vi "Untitled 1.vi"() -> ()   [LabVIEW 2015]
uses:
  Setting_Control_Main Action.ctl
  <vilib>/Utility/miscctls.llb/LVPositionTypeDef.ctl
  <vilib>/ptbypt/NI_PtbyPt.lvlib
panel:
  in  "Boolean":bool
  out "Array":T1[](array[typedef])=[enum."二、動作-單次取像", enum."三、動作-連續取像"]
  out "Setting Action":T1
  in  "Tab Control":enum32{"設定", "Match參數", "找邊參數", "找圓參數"}(tab)
  in  "功能選擇":enum16{"Pattern", "Match", "找邊", "找圓"}(ring)
  in  "匯入圖片":bool
  in  "確認檢測項目":bool
  in  "Cluster":T2
  out "Pattern":T3(plugin-control)
  out "Image":T3(plugin-control)
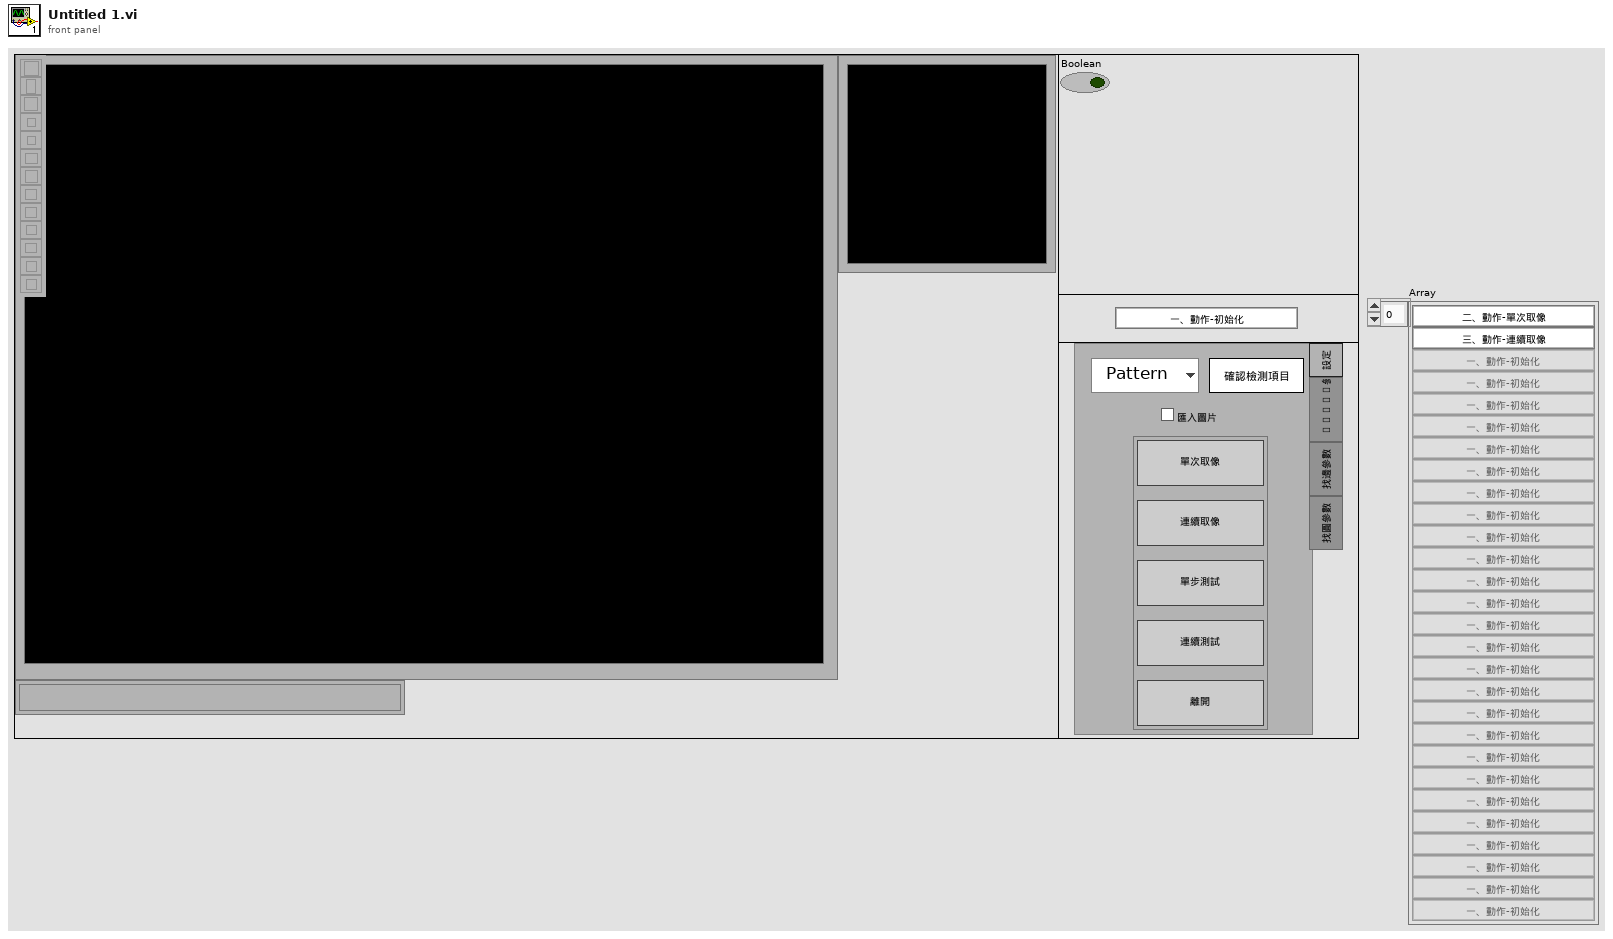
[diagram p1: front panel]
types:
  T1 = typedef "Setting_Control_Main Action.ctl" = enum16{"一、動作-初始化", "二、動作-單次取像", "三、動作-連續取像", "四、動作-單步測試", "五、動作-連續測試", "六、動作-離開", "1.0 功能-IO控制", "       1.1 IO-初始化", "       1.2 Set Point(EOT On)", "       1.3Set Point(EOT Off)", "       1.4Get Point(SOT)", "2.0功能-相機控制", "       2.1相機-初始化", "       2.2相機-取像", "       2.3相機-關閉", "3.0功能-影像控制", "       3.1影像-初始化", "       3.2影像-更新影像", "       3.3影像-儲存影像", "4.0功能-檢測", "       4.1檢測-初始化", "      4.2浪代-浪代", "             4.2.1浪代-Pattern", "             4.2.2浪代-Match", "             4.2.3檢測-找邊", "             4.2.4檢測-找圓", "5.0功能-檔案", "       5.1檔案-初始化", "       5.2檔案-儲存檔案", "       5.3檔案-開啟檔案", "       5.4檔案-匯入檔案", "6.0 錯誤", "7.0等待", "       7.1等待(計算時間)", "8.0離開", "9.0功能-機台驗證", "      9.1機台驗證-初始化", "      9.2機台驗證-檢測", "10.0對話視窗", "11.光源控制", "       11.1光源控制-初始化", "       11.2光源控制-光源開啟", "       11.3光源控制-光源關閉", "       11.4光源控制-通訊關閉"}
  T2 = cluster{"二、動作-單次取像":bool, "三、動作-連續取像":bool, "四、動作-單步測試":bool, "五、動作-連續測試":bool, "六、動作-離開":bool}
  T3 = typedef "IMAQ Image.ctl" = refnum<image>
  T4 = typedef "LVPositionTypeDef.ctl" = cluster{"Left":i32, "Top":i32}
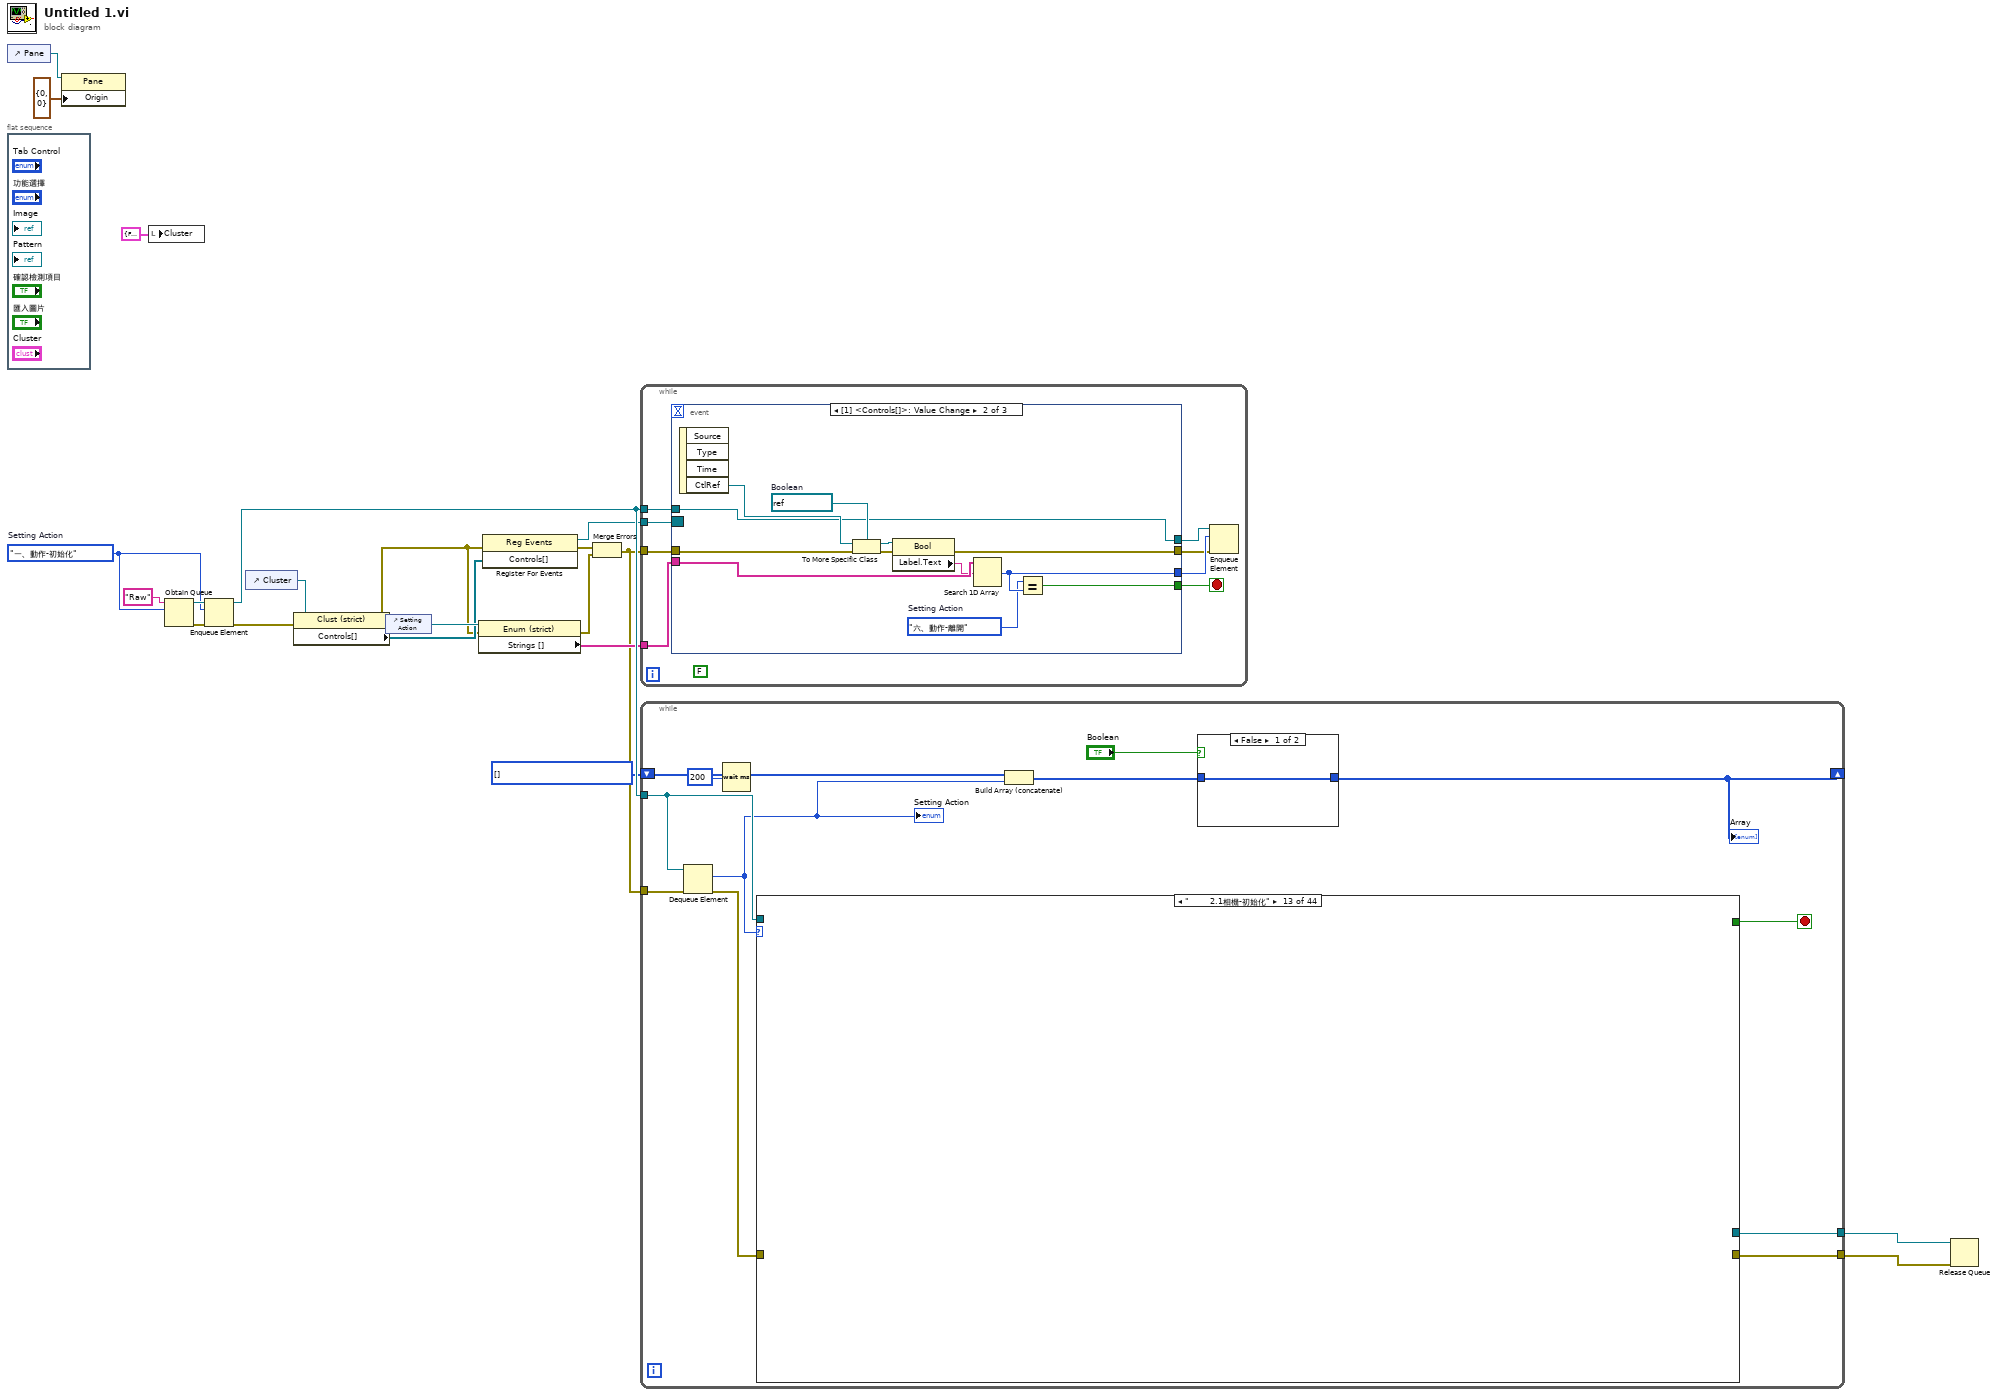
[diagram p0: block diagram]
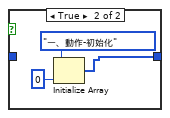
[diagram p2: hidden frame]
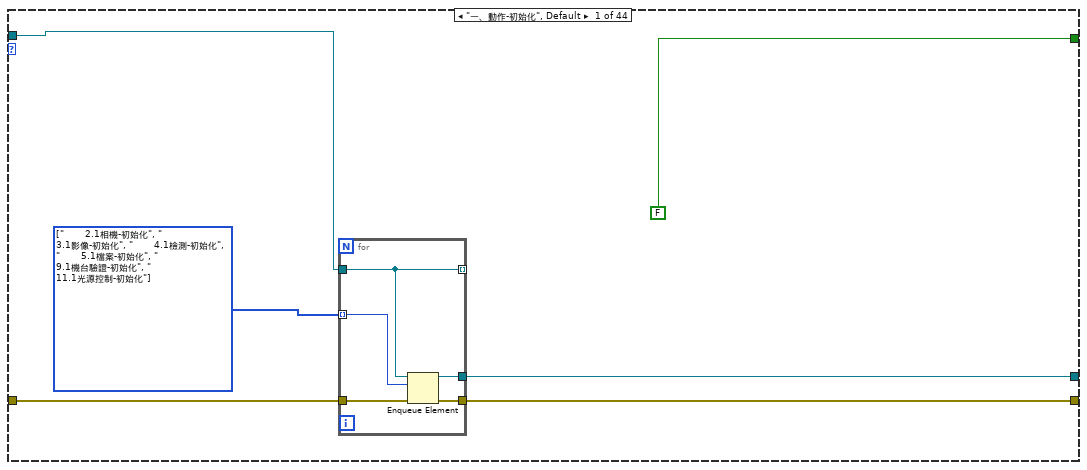
[diagram p3: hidden frame]
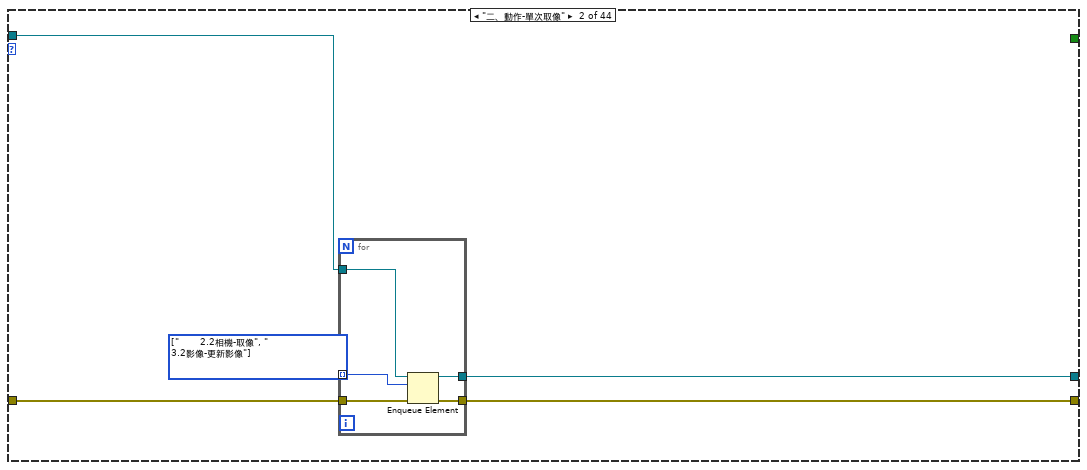
[diagram p4: hidden frame]
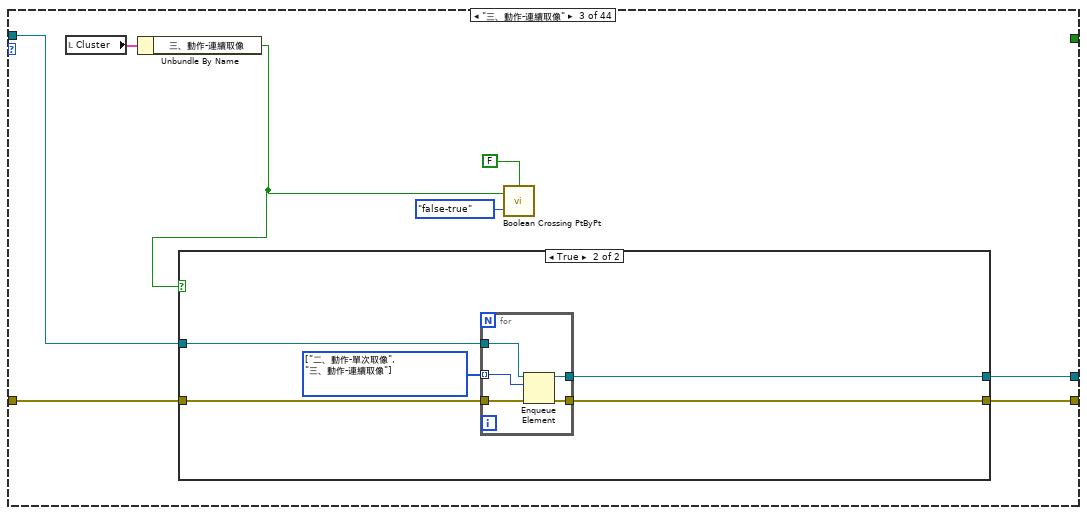
[diagram p5: hidden frame]
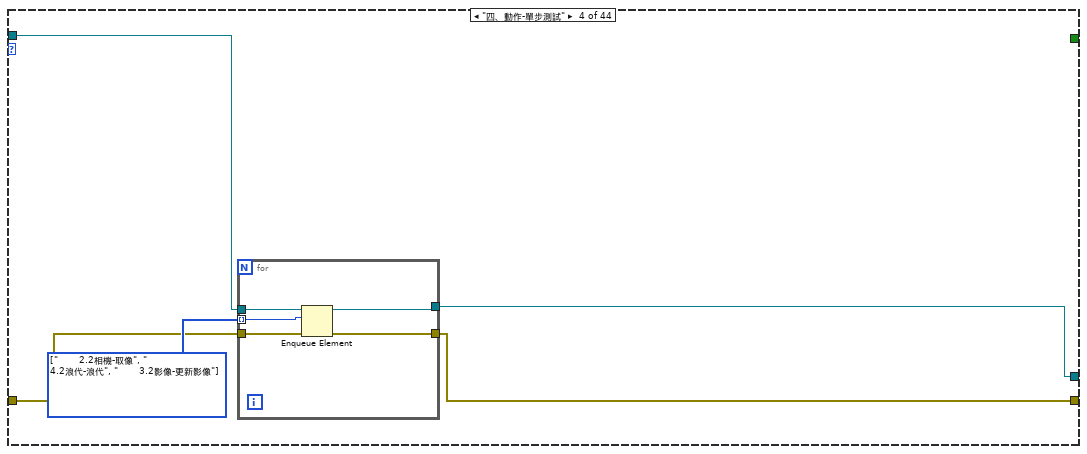
[diagram p7: hidden frame]
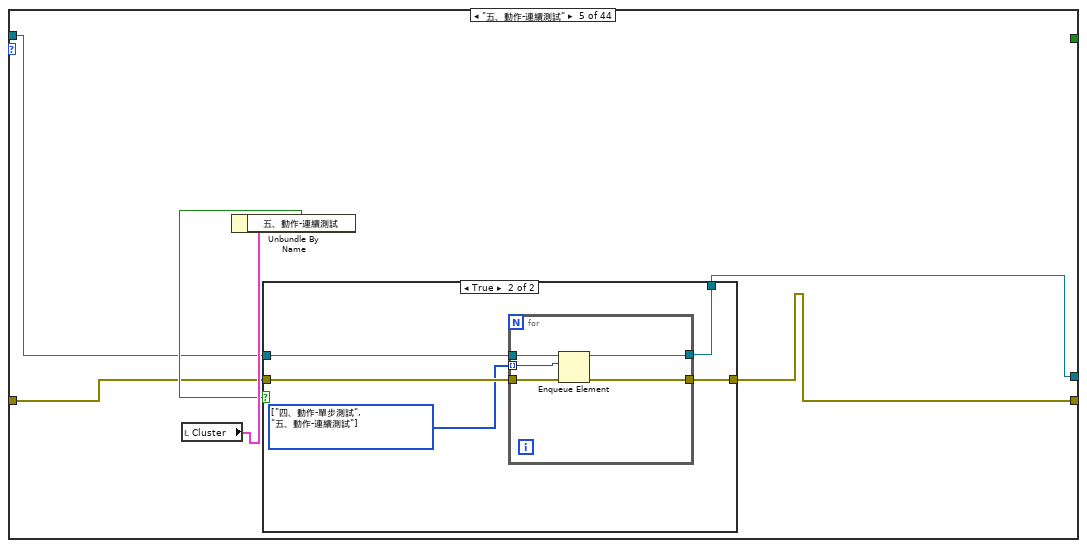
[diagram p8: hidden frame]
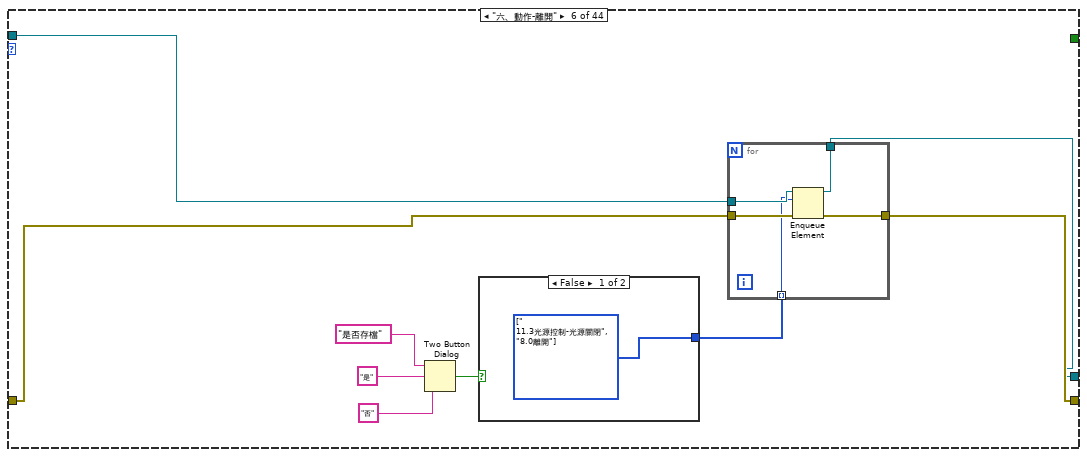
[diagram p10: hidden frame]
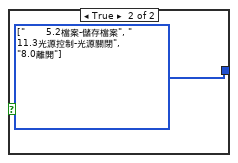
[diagram p11: hidden frame]
diagram:
  w2 = T1[] [] items=["一、動作-初始化", "二、動作-單次取像", "三、動作-連續取像", "四、動作-單步測試", "五、動作-連續測試", "六、動作-離開", "1.0 功能-IO控制", "       1.1 IO-初始化", "       1.2 Set Point(EOT On)", "       1.3Set Point(EOT Off)", "       1.4Get Point(SOT)", "2.0功能-相機控制", "       2.1相機-初始化", "       2.2相機-取像", "       2.3相機-關閉", "3.0功能-影像控制", "       3.1影像-初始化", "       3.2影像-更新影像", "       3.3影像-儲存影像", "4.0功能-檢測", "       4.1檢測-初始化", "      4.2浪代-浪代", "             4.2.1浪代-Pattern", "             4.2.2浪代-Match", "             4.2.3檢測-找邊", "             4.2.4檢測-找圓", "5.0功能-檔案", "       5.1檔案-初始化", "       5.2檔案-儲存檔案", "       5.3檔案-開啟檔案", "       5.4檔案-匯入檔案", "6.0 錯誤", "7.0等待", "       7.1等待(計算時間)", "8.0離開", "9.0功能-機台驗證", "      9.1機台驗證-初始化", "      9.2機台驗證-檢測", "10.0對話視窗", "11.光源控制", "       11.1光源控制-初始化", "       11.2光源控制-光源開啟", "       11.3光源控制-光源關閉", "       11.4光源控制-通訊關閉"]
  w11 = Setting_Control_Main_Action."一、動作-初始化"  # Setting Action
  n1 = control-ref of="Pane"() -> (w13:refnum<vi>)
  n2 = flat-sequence {
    frame #0 {
    }
  }
  n3 = property class="Pane"(reference=w13, "Origin"=T4 {"Left"=0, "Top"=0} ("Position")) -> ()  [unwired: 1 in, 2 out]
  n4 = local write "Cluster"(T2 {"二、動作-單次取像"=FALSE, "三、動作-連續取像"=FALSE, "四、動作-單步測試"=FALSE, "五、動作-連續測試"=FALSE, "六、動作-離開"=FALSE} ("Cluster")) -> ()
  n5 = Obtain Queue(name (unnamed)="Raw", element data type=w11) -> (queue out=w21:refnum<queue>, error out=w10:errorcluster)  [unwired: 3 in, 1 out]
  n6 = Enqueue Element(queue=w21, element=w11, error in (no error)=w10) -> (queue out=w19:refnum<queue>, error out=w9:errorcluster)  [unwired: 1 in, 1 out]
  n7 = control-ref of="Cluster"() -> (w15:refnum<vi>)
  n8 = property class="Clust (strict)"(reference=w15, error in=w9) -> (error out=w8:errorcluster, "Controls[]"=w14:refnum<vi>[])  [unwired: 1 out]
  n9 = control-ref of="Setting Action"() -> (w17:refnum<vi>)
  n10 = property class="Enum (strict)"(reference=w17, error in=w8) -> (error out=w6:errorcluster, "Strings []"=w16:string[])  [unwired: 1 out]
  n11 = register-events(error in=w8, w14) -> (reference out=w18:refnum<event-registration>, error out=w7:errorcluster)  [unwired: 1 in]
  n12 = Merge Errors(w7, w6) -> (w5:errorcluster)
  n13 = while {
    tunnel: w19 -> [w29]
    tunnel: w18 -> [w28]
    tunnel: w16 -> [w27]
    tunnel: w5 -> [w23]
    stop <- w26 stop-if-true
    (unwired) FALSE
    n14 = event shown="[1] <Controls[]>: Value Change" {
      selector: w28 -> [_ _ _]
      dyn-events: _ -> [_ _ _]
      timeout: _ -> [_ _ _]
      tunnel: [w31 w37 w45] -> w25
      tunnel: w29 -> [w31 w37 w47]
      tunnel: w27 -> [_ w40 _]
      tunnel: [_ w38 _] -> w26
      tunnel: [_ w36 w46] -> w24
      tunnel: w23 -> [w30 w34 w44]
      tunnel: [w30 w32 _] -> w22
      event Timeout {
        n15 = event-data() -> ()  [unwired: 1 in, 3 out]
      }
      event Value Change {
        w35 = Setting_Control_Main_Action."六、動作-離開"  # Setting Action
        w43 = refnum<vi> refnum  # Boolean
        n16 = event-data() -> ("CtlRef"=w41:refnum<vi>)  [unwired: 1 in, 3 out]
        n17 = To More Specific Class(target class=w43, reference=w41, error in=w34) -> (specific class reference=w42:refnum<vi>, error out=w33:errorcluster)
        n18 = property class="Bool"(reference=w42, error in=w33) -> (error out=w32:errorcluster, "Label.Text"=w39:string)  [unwired: 1 out]
        n19 = Search 1D Array(1D array=w40, element=w39) -> (index of element=w36:i32)  [unwired: 1 in]
        n20 = Equal?(x=w35, y=w36) -> (x = y?=w38:bool)
      }
      event "確認檢測項目": Value Change {
        n21 = event-data() -> ()  [unwired: 1 in, 4 out]
        n22 = local read "功能選擇"() -> (w48:enum16{"Pattern", "Match", "找邊", "找圓"})
        n23 = case shown="\"Match\"" w48 {
          tunnel: w47 -> [w51 w54 w57 w60]
          tunnel: [w51 w54 w57 w60] -> w45
          tunnel: w44 -> [w50 w53 w56 w59]
          tunnel: [w50 w53 w56 w59] -> _
          tunnel: [Setting_Control_Main_Action."             4.2.1浪代-Pattern" ("Set action") Setting_Control_Main_Action."             4.2.2浪代-Match" ("Set action") Setting_Control_Main_Action."             4.2.3檢測-找邊" ("Set action") Setting_Control_Main_Action."             4.2.4檢測-找圓" ("Set action")] -> w46
          frame "Pattern", Default {
          }
          frame "Match" {
          }
          frame "找邊" {
          }
          frame "找圓" {
          }
        }
      }
    }
    n24 = Enqueue Element(queue=w25, element=w24, error in (no error)=w22) -> ()  [unwired: 1 in, 3 out]
  }
  n25 = while {
    tunnel: w19 -> [w69]
    tunnel: w5 -> [w70]
    tunnel: [w61] -> w4
    tunnel: [w67] -> w3
    shift-right: [w62] -> _
    shift-left: w2 -> [w65]
    stop <- w72 stop-if-true
    n26 = Dequeue Element(queue=w69, error in (no error)=w70) -> (element=w66:T1, error out=w68:errorcluster)  [unwired: 1 in, 2 out]
    "Setting Action" <- w66
    n27 = Wait (ms)(milliseconds to wait=u32 200) -> ()  [unwired: 1 out]
    n28 = case shown="\"       2.1相機-初始化\"" w66 {
      tunnel: [FALSE _ _ _ _ _ _ _ _ _ _ _ _ _ _ _ _ _ _ _ _ _ _ _ _ _ _ _ _ _ _ _ _ _ TRUE _ _ _ _ _ _ _ _ _] -> w72
      tunnel: [w81 w89 w102 w118 w128 w146 _ _ _ _ _ _ _ _ _ _ _ _ _ _ _ _ _ _ _ _ _ _ _ _ _ _ _ _ _ _ _ _ _ _ _ _ _ _] -> w61
      tunnel: w69 -> [w80 w91 w105 w121 w131 w149 _ _ _ _ _ _ _ _ _ _ _ _ _ _ _ _ _ _ _ _ _ _ _ _ _ _ _ _ _ _ _ _ _ _ _ _ _ _]
      tunnel: w68 -> [w79 w90 w103 w120 w130 w148 _ _ _ _ _ _ _ _ _ _ _ _ _ _ _ _ _ _ _ _ _ _ _ _ _ _ _ _ _ _ _ _ _ _ _ _ _ _]
      tunnel: [w77 w88 w104 w119 w129 w147 _ _ _ _ _ _ _ _ _ _ _ _ _ _ _ _ _ _ _ _ _ _ _ _ _ _ _ _ _ _ _ _ _ _ _ _ _ _] -> w67
      frame "一、動作-初始化", Default {
        w78 = T1[] [enum."       2.1相機-初始化", enum."       3.1影像-初始化", enum."       4.1檢測-初始化", enum."       5.1檔案-初始化", enum."      9.1機台驗證-初始化", enum."       11.1光源控制-初始化"] items=["一、動作-初始化", "二、動作-單次取像", "三、動作-連續取像", "四、動作-單步測試", "五、動作-連續測試", "六、動作-離開", "1.0 功能-IO控制", "       1.1 IO-初始化", "       1.2 Set Point(EOT On)", "       1.3Set Point(EOT Off)", "       1.4Get Point(SOT)", "2.0功能-相機控制", "       2.1相機-初始化", "       2.2相機-取像", "       2.3相機-關閉", "3.0功能-影像控制", "       3.1影像-初始化", "       3.2影像-更新影像", "       3.3影像-儲存影像", "4.0功能-檢測", "       4.1檢測-初始化", "      4.2浪代-浪代", "             4.2.1浪代-Pattern", "             4.2.2浪代-Match", "             4.2.3檢測-找邊", "             4.2.4檢測-找圓", "5.0功能-檔案", "       5.1檔案-初始化", "       5.2檔案-儲存檔案", "       5.3檔案-開啟檔案", "       5.4檔案-匯入檔案", "6.0 錯誤", "7.0等待", "       7.1等待(計算時間)", "8.0離開", "9.0功能-機台驗證", "      9.1機台驗證-初始化", "      9.2機台驗證-檢測", "10.0對話視窗", "11.光源控制", "       11.1光源控制-初始化", "       11.2光源控制-光源開啟", "       11.3光源控制-光源關閉", "       11.4光源控制-通訊關閉"]
        n29 = for {
          tunnel: [w83] -> _ mode=indexing
          tunnel: w79 -> [w87]
          tunnel: [w86] -> w77
          tunnel: [w85] -> w81
          tunnel: w78 -> [w84] mode=indexing
          tunnel: w80 -> [w83]
          n30 = Enqueue Element(queue=w83, element=w84, error in (no error)=w87) -> (queue out=w85:refnum<queue>, error out=w86:errorcluster)  [unwired: 1 in, 1 out]
        }
      }
      frame "二、動作-單次取像" {
        w92 = T1[] [enum."       2.2相機-取像", enum."       3.2影像-更新影像"] items=["一、動作-初始化", "二、動作-單次取像", "三、動作-連續取像", "四、動作-單步測試", "五、動作-連續測試", "六、動作-離開", "1.0 功能-IO控制", "       1.1 IO-初始化", "       1.2 Set Point(EOT On)", "       1.3Set Point(EOT Off)", "       1.4Get Point(SOT)", "2.0功能-相機控制", "       2.1相機-初始化", "       2.2相機-取像", "       2.3相機-關閉", "3.0功能-影像控制", "       3.1影像-初始化", "       3.2影像-更新影像", "       3.3影像-儲存影像", "4.0功能-檢測", "       4.1檢測-初始化", "      4.2浪代-浪代", "             4.2.1浪代-Pattern", "             4.2.2浪代-Match", "             4.2.3檢測-找邊", "             4.2.4檢測-找圓", "5.0功能-檔案", "       5.1檔案-初始化", "       5.2檔案-儲存檔案", "       5.3檔案-開啟檔案", "       5.4檔案-匯入檔案", "6.0 錯誤", "7.0等待", "       7.1等待(計算時間)", "8.0離開", "9.0功能-機台驗證", "      9.1機台驗證-初始化", "      9.2機台驗證-檢測", "10.0對話視窗", "11.光源控制", "       11.1光源控制-初始化", "       11.2光源控制-光源開啟", "       11.3光源控制-光源關閉", "       11.4光源控制-通訊關閉"]
        n31 = for {
          tunnel: w91 -> [w97]
          tunnel: w90 -> [w96]
          tunnel: [w95] -> w88
          tunnel: [w94] -> w89
          tunnel: w92 -> [w93] mode=indexing
          n32 = Enqueue Element(queue=w97, element=w93, error in (no error)=w96) -> (queue out=w94:refnum<queue>, error out=w95:errorcluster)  [unwired: 1 in, 1 out]
        }
      }
      frame "三、動作-連續取像" {
        n33 = local read "Cluster"() -> (w101:T2)
        n34 = Unbundle By Name(w101) -> ("三、動作-連續取像"=w98:bool)
        n35 = case shown="True" w98 {
          tunnel: w105 -> [w107 w111]
          tunnel: w103 -> [w106 w110]
          tunnel: [w107 w109] -> w102
          tunnel: [w106 w108] -> w104
          frame False {
          }
          frame True {
            w112 = T1[] [enum."二、動作-單次取像", enum."三、動作-連續取像"] items=["一、動作-初始化", "二、動作-單次取像", "三、動作-連續取像", "四、動作-單步測試", "五、動作-連續測試", "六、動作-離開", "1.0 功能-IO控制", "       1.1 IO-初始化", "       1.2 Set Point(EOT On)", "       1.3Set Point(EOT Off)", "       1.4Get Point(SOT)", "2.0功能-相機控制", "       2.1相機-初始化", "       2.2相機-取像", "       2.3相機-關閉", "3.0功能-影像控制", "       3.1影像-初始化", "       3.2影像-更新影像", "       3.3影像-儲存影像", "4.0功能-檢測", "       4.1檢測-初始化", "      4.2浪代-浪代", "             4.2.1浪代-Pattern", "             4.2.2浪代-Match", "             4.2.3檢測-找邊", "             4.2.4檢測-找圓", "5.0功能-檔案", "       5.1檔案-初始化", "       5.2檔案-儲存檔案", "       5.3檔案-開啟檔案", "       5.4檔案-匯入檔案", "6.0 錯誤", "7.0等待", "       7.1等待(計算時間)", "8.0離開", "9.0功能-機台驗證", "      9.1機台驗證-初始化", "      9.2機台驗證-檢測", "10.0對話視窗", "11.光源控制", "       11.1光源控制-初始化", "       11.2光源控制-光源開啟", "       11.3光源控制-光源關閉", "       11.4光源控制-通訊關閉"]
            n36 = for {
              tunnel: [w117] -> w108
              tunnel: [w116] -> w109
              tunnel: w112 -> [w115] mode=indexing
              tunnel: w111 -> [w114]
              tunnel: w110 -> [w113]
              n37 = Enqueue Element(queue=w114, element=w115, error in (no error)=w113) -> (queue out=w116:refnum<queue>, error out=w117:errorcluster)  [unwired: 1 in, 1 out]
            }
          }
        }
        n38 = call <vilib>:"Boolean Crossing PtByPt.vi"("initialize"=FALSE, "direction"=enum16{"either", "false-true", "true-false"}."false-true", "input"=w98) -> ()  [unwired: 1 out]
      }
      frame "四、動作-單步測試" {
        w122 = T1[] [enum."       2.2相機-取像", enum."      4.2浪代-浪代", enum."       3.2影像-更新影像"] items=["一、動作-初始化", "二、動作-單次取像", "三、動作-連續取像", "四、動作-單步測試", "五、動作-連續測試", "六、動作-離開", "1.0 功能-IO控制", "       1.1 IO-初始化", "       1.2 Set Point(EOT On)", "       1.3Set Point(EOT Off)", "       1.4Get Point(SOT)", "2.0功能-相機控制", "       2.1相機-初始化", "       2.2相機-取像", "       2.3相機-關閉", "3.0功能-影像控制", "       3.1影像-初始化", "       3.2影像-更新影像", "       3.3影像-儲存影像", "4.0功能-檢測", "       4.1檢測-初始化", "      4.2浪代-浪代", "             4.2.1浪代-Pattern", "             4.2.2浪代-Match", "             4.2.3檢測-找邊", "             4.2.4檢測-找圓", "5.0功能-檔案", "       5.1檔案-初始化", "       5.2檔案-儲存檔案", "       5.3檔案-開啟檔案", "       5.4檔案-匯入檔案", "6.0 錯誤", "7.0等待", "       7.1等待(計算時間)", "8.0離開", "9.0功能-機台驗證", "      9.1機台驗證-初始化", "      9.2機台驗證-檢測", "10.0對話視窗", "11.光源控制", "       11.1光源控制-初始化", "       11.2光源控制-光源開啟", "       11.3光源控制-光源關閉", "       11.4光源控制-通訊關閉"]
        n39 = for {
          tunnel: w121 -> [w127]
          tunnel: w120 -> [w126]
          tunnel: [w125] -> w118
          tunnel: [w124] -> w119
          tunnel: w122 -> [w123] mode=indexing
          n40 = Enqueue Element(queue=w127, element=w123, error in (no error)=w126) -> (queue out=w125:refnum<queue>, error out=w124:errorcluster)  [unwired: 1 in, 1 out]
        }
      }
      frame "五、動作-連續測試" {
        n41 = local read "Cluster"() -> (w133:T2)
        n42 = Unbundle By Name(w133) -> ("五、動作-連續測試"=w132:bool)
        n43 = case shown="True" w132 {
          tunnel: w131 -> [w135 w140]
          tunnel: w130 -> [w134 w139]
          tunnel: [w135 w138] -> w128
          tunnel: [w134 w137] -> w129
          frame False {
          }
          frame True {
            w136 = T1[] [enum."四、動作-單步測試", enum."五、動作-連續測試"] items=["一、動作-初始化", "二、動作-單次取像", "三、動作-連續取像", "四、動作-單步測試", "五、動作-連續測試", "六、動作-離開", "1.0 功能-IO控制", "       1.1 IO-初始化", "       1.2 Set Point(EOT On)", "       1.3Set Point(EOT Off)", "       1.4Get Point(SOT)", "2.0功能-相機控制", "       2.1相機-初始化", "       2.2相機-取像", "       2.3相機-關閉", "3.0功能-影像控制", "       3.1影像-初始化", "       3.2影像-更新影像", "       3.3影像-儲存影像", "4.0功能-檢測", "       4.1檢測-初始化", "      4.2浪代-浪代", "             4.2.1浪代-Pattern", "             4.2.2浪代-Match", "             4.2.3檢測-找邊", "             4.2.4檢測-找圓", "5.0功能-檔案", "       5.1檔案-初始化", "       5.2檔案-儲存檔案", "       5.3檔案-開啟檔案", "       5.4檔案-匯入檔案", "6.0 錯誤", "7.0等待", "       7.1等待(計算時間)", "8.0離開", "9.0功能-機台驗證", "      9.1機台驗證-初始化", "      9.2機台驗證-檢測", "10.0對話視窗", "11.光源控制", "       11.1光源控制-初始化", "       11.2光源控制-光源開啟", "       11.3光源控制-光源關閉", "       11.4光源控制-通訊關閉"]
            n44 = for {
              tunnel: w140 -> [w145]
              tunnel: w139 -> [w144]
              tunnel: [w143] -> w138
              tunnel: [w142] -> w137
              tunnel: w136 -> [w141] mode=indexing
              n45 = Enqueue Element(queue=w145, element=w141, error in (no error)=w144) -> (queue out=w143:refnum<queue>, error out=w142:errorcluster)  [unwired: 1 in, 1 out]
            }
          }
        }
      }
      frame "六、動作-離開" {
        n46 = Two Button Dialog(message="是否存檔", 1:"否" ("F button name (\"Cancel\")"), 2:"是" ("T button name (\"OK\")")) -> (T button?=w154:bool)
        n47 = case shown="False" w154 {
          tunnel: [w155 w156] -> w150
          frame False {
            w155 = T1[] [enum."       11.3光源控制-光源關閉", enum."8.0離開"] items=["一、動作-初始化", "二、動作-單次取像", "三、動作-連續取像", "四、動作-單步測試", "五、動作-連續測試", "六、動作-離開", "1.0 功能-IO控制", "       1.1 IO-初始化", "       1.2 Set Point(EOT On)", "       1.3Set Point(EOT Off)", "       1.4Get Point(SOT)", "2.0功能-相機控制", "       2.1相機-初始化", "       2.2相機-取像", "       2.3相機-關閉", "3.0功能-影像控制", "       3.1影像-初始化", "       3.2影像-更新影像", "       3.3影像-儲存影像", "4.0功能-檢測", "       4.1檢測-初始化", "      4.2浪代-浪代", "             4.2.1浪代-Pattern", "             4.2.2浪代-Match", "             4.2.3檢測-找邊", "             4.2.4檢測-找圓", "5.0功能-檔案", "       5.1檔案-初始化", "       5.2檔案-儲存檔案", "       5.3檔案-開啟檔案", "       5.4檔案-匯入檔案", "6.0 錯誤", "7.0等待", "       7.1等待(計算時間)", "8.0離開", "9.0功能-機台驗證", "      9.1機台驗證-初始化", "      9.2機台驗證-檢測", "10.0對話視窗", "11.光源控制", "       11.1光源控制-初始化", "       11.2光源控制-光源開啟", "       11.3光源控制-光源關閉", "       11.4光源控制-通訊關閉"]
          }
          frame True {
            w156 = T1[] [enum."       5.2檔案-儲存檔案", enum."       11.3光源控制-光源關閉", enum."8.0離開"] items=["一、動作-初始化", "二、動作-單次取像", "三、動作-連續取像", "四、動作-單步測試", "五、動作-連續測試", "六、動作-離開", "1.0 功能-IO控制", "       1.1 IO-初始化", "       1.2 Set Point(EOT On)", "       1.3Set Point(EOT Off)", "       1.4Get Point(SOT)", "2.0功能-相機控制", "       2.1相機-初始化", "       2.2相機-取像", "       2.3相機-關閉", "3.0功能-影像控制", "       3.1影像-初始化", "       3.2影像-更新影像", "       3.3影像-儲存影像", "4.0功能-檢測", "       4.1檢測-初始化", "      4.2浪代-浪代", "             4.2.1浪代-Pattern", "             4.2.2浪代-Match", "             4.2.3檢測-找邊", "             4.2.4檢測-找圓", "5.0功能-檔案", "       5.1檔案-初始化", "       5.2檔案-儲存檔案", "       5.3檔案-開啟檔案", "       5.4檔案-匯入檔案", "6.0 錯誤", "7.0等待", "       7.1等待(計算時間)", "8.0離開", "9.0功能-機台驗證", "      9.1機台驗證-初始化", "      9.2機台驗證-檢測", "10.0對話視窗", "11.光源控制", "       11.1光源控制-初始化", "       11.2光源控制-光源開啟", "       11.3光源控制-光源關閉", "       11.4光源控制-通訊關閉"]
          }
        }
        n48 = for {
          tunnel: w149 -> [w161]
          tunnel: w148 -> [w160]
          tunnel: [w159] -> w146
          tunnel: [w158] -> w147
          tunnel: w150 -> [w157] mode=indexing
          n49 = Enqueue Element(queue=w161, element=w157, error in (no error)=w160) -> (queue out=w159:refnum<queue>, error out=w158:errorcluster)  [unwired: 1 in, 1 out]
        }
      }
      frame "1.0 功能-IO控制" {
      }
      frame "       1.1 IO-初始化" {
      }
      frame "       1.2 Set Point(EOT On)" {
      }
      frame "       1.3Set Point(EOT Off)" {
      }
      frame "       1.4Get Point(SOT)" {
      }
      frame "2.0功能-相機控制" {
      }
      frame "       2.1相機-初始化" {
      }
      frame "       2.2相機-取像" {
      }
      frame "       2.3相機-關閉" {
      }
      frame "3.0功能-影像控制" {
      }
      frame "       3.1影像-初始化" {
      }
      frame "       3.2影像-更新影像" {
      }
      frame "       3.3影像-儲存影像" {
      }
      frame "4.0功能-檢測" {
      }
      frame "       4.1檢測-初始化" {
      }
      frame "      4.2浪代-浪代" {
      }
      frame "             4.2.1浪代-Pattern" {
      }
      frame "             4.2.2浪代-Match" {
      }
      frame "             4.2.3檢測-找邊" {
      }
      frame "             4.2.4檢測-找圓" {
      }
      frame "5.0功能-檔案" {
      }
      frame "       5.1檔案-初始化" {
      }
      frame "       5.2檔案-儲存檔案" {
      }
      frame "       5.3檔案-開啟檔案" {
      }
      frame "       5.4檔案-匯入檔案" {
      }
      frame "6.0 錯誤" {
      }
      frame "7.0等待" {
      }
      frame "       7.1等待(計算時間)" {
      }
      frame "8.0離開" {
      }
      frame "9.0功能-機台驗證" {
      }
      frame "      9.1機台驗證-初始化" {
      }
      frame "      9.2機台驗證-檢測" {
      }
      frame "10.0對話視窗" {
      }
      frame "11.光源控制" {
      }
      frame "       11.1光源控制-初始化" {
      }
      frame "       11.2光源控制-光源開啟" {
      }
      frame "       11.3光源控制-光源關閉" {
      }
      frame "       11.4光源控制-通訊關閉" {
      }
    }
    n50 = Build Array (concatenate)(w65, w66) -> (w63:T1[])
    n51 = case shown="False" "Boolean" {
      tunnel: w63 -> [w73 _]
      tunnel: [w73 w76] -> w62
      frame False {
      }
      frame True {
        n52 = Initialize Array(Setting_Control_Main_Action."一、動作-初始化" ("Setting Action 2"), 0 ("dimension size")) -> (w76:T1[])
      }
    }
    "Array" <- w62
  }
  n53 = Release Queue(queue=w4, error in (no error)=w3) -> ()  [unwired: 1 in, 3 out]
